vi "TEMPLATE.vi"(7 "Sender":refnum<class "Sender.lvclass">, 11 "TEMPLATE in":refnum<class "TEMPLATE.lvclass">) -> (3 "TEMPLATE out":refnum<class "TEMPLATE.lvclass">)   [LabVIEW 2020, in "_Template.lvlib" / "Templates.lvlib" / "TEMPLATE Msg.lvlib" / "TEMPLATE.lvclass"]
uses:
  TEMPLATE.lvclass
  jettl/jettl/Sender/Sender/Sender.lvclass
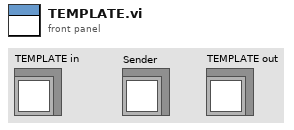
[diagram p1: front panel]
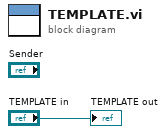
[diagram p0: block diagram]
diagram:
  "TEMPLATE out" <- "TEMPLATE in"
